vi "Module Pre-Build.vi"(6 "action":enum16{"nothing", "pre-build", "post-build"}(ring), 7 "Post-build parameters":T8 {"Build Version Info"."Build Date/Time" format="%<%H:%M:%S\n%d/%m/%Y>T"}, 8 "error in":errorcluster, 11 "Build Parameters in":T1={"Build File"=path "", "File Format Version"=0, "Build Parameters v0.0"={"Project Root"=path "", "Build Root"=path "", "Source Root"=path "", "Namespace"="", "Overwrite Existing Files?"=FALSE, "Top Level VIs"=[], "Dynamic VIs"=[], "Exclude Lib Dirs from Build (None)"=[], "Destinations"=[]}, "Extra Parameters v1.0"={"Log File"=path "", "Include Hidden VIs"=FALSE, "Include Help Files"=FALSE, "Help File Dir"=path "", "Include Shared Libs"=TRUE, "Shared Lib Dir"=path "", "Include External Subrs"=TRUE, "External Subr Dir"=path "", "Support Files"=[], "EXE Icon File"=path "", "NewBuildRootDir"=FALSE, "UnsavedChangesMsgBox"=FALSE, "Ambiguous VIs Dest Dir"=path "", "Pre-build VI"=path "", "Post-build VI"=path "", "Revision File"=path "", "Version VI Name"="", "Version Ctrl Name"="", "Default Password"="", "RemovePolyVIsAndTDs"=FALSE, "Call-Back VIs"=[], "Allow CBVI & BH overlap"=FALSE, "Namespace convention"=enum."OpenG (suffix)", "Exe.AppFlags"=0, "Exe.LVRT Res Flags"=0}, "VI Property Specs"=[]} {"File Format Version" format="%.0x"; "Extra Parameters v1.0"."Exe.LVRT Res Flags" format="%.0x"; "Extra Parameters v1.0"."Exe.AppFlags" format="%.0x"}) -> (0 "error out":errorcluster, 1 "error type":enum16{"fatal", "non-fatal", "warning"}(ring), 3 "Build Parameters out":T1={"Build File"=path "", "File Format Version"=0, "Build Parameters v0.0"={"Project Root"=path "", "Build Root"=path "", "Source Root"=path "", "Namespace"="", "Overwrite Existing Files?"=FALSE, "Top Level VIs"=[], "Dynamic VIs"=[], "Exclude Lib Dirs from Build (None)"=[], "Destinations"=[]}, "Extra Parameters v1.0"={"Log File"=path "", "Include Hidden VIs"=FALSE, "Include Help Files"=FALSE, "Help File Dir"=path "", "Include Shared Libs"=TRUE, "Shared Lib Dir"=path "", "Include External Subrs"=TRUE, "External Subr Dir"=path "", "Support Files"=[], "EXE Icon File"=path "", "NewBuildRootDir"=FALSE, "UnsavedChangesMsgBox"=FALSE, "Ambiguous VIs Dest Dir"=path "", "Pre-build VI"=path "", "Post-build VI"=path "", "Revision File"=path "", "Version VI Name"="", "Version Ctrl Name"="", "Default Password"="", "RemovePolyVIsAndTDs"=FALSE, "Call-Back VIs"=[], "Allow CBVI & BH overlap"=FALSE, "Namespace convention"=enum."OpenG (suffix)", "Exe.AppFlags"=0, "Exe.LVRT Res Flags"=0}, "VI Property Specs"=[]} {"File Format Version" format="%.0x"; "Extra Parameters v1.0"."Exe.LVRT Res Flags" format="%.0x"; "Extra Parameters v1.0"."Exe.AppFlags" format="%.0x"})   [LabVIEW 2011]
doc: "Use this VI Template to create a custom Pre-/Post-Build VI."
uses:
  <userlib>/_OpenG.lib/builder_api/ogb_api.llb/Post-build Actual Parameters__ogb_api.ctl
  <userlib>/_OpenG.lib/builder_api/ogb_api.llb/VI Build Info__ogb_api.ctl
  <userlib>/_OpenG.lib/builder_api/ogb_api.llb/Non-VI Resource Copy Info__ogb_api.ctl
  <userlib>/_OpenG.lib/builder_api/ogb_api.llb/Link Type - Enum__ogb_api.ctl
  <userlib>/_OpenG.lib/builder_api/ogb_api.llb/Version Info Cluster__ogb_api.ctl
  <userlib>/_OpenG.lib/builder_api/ogb_api.llb/Build Parameters__ogb_api.ctl
  <userlib>/_OpenG.lib/builder_api/ogb_api.llb/Build Parameters Cluster v0.0__ogb_api.ctl
  <userlib>/_OpenG.lib/builder_api/ogb_api.llb/Source Dir and Destination Cluster__ogb_api.ctl
  <userlib>/_OpenG.lib/builder_api/ogb_api.llb/Extra Build Parameters Cluster v1.0__ogb_api.ctl
  <userlib>/_OpenG.lib/builder_api/ogb_api.llb/Support Files Info Cluster__ogb_api.ctl
  <userlib>/_OpenG.lib/builder_api/ogb_api.llb/Namespasing Convention__ogb_api.ctl
  <userlib>/_OpenG.lib/builder_api/ogb_api.llb/VI Property Specifiers Info Cluster__ogb_api.ctl
  <userlib>/_OpenG.lib/file/file.llb/Append Path to Root if Relative - Scalar__ogtk.vi
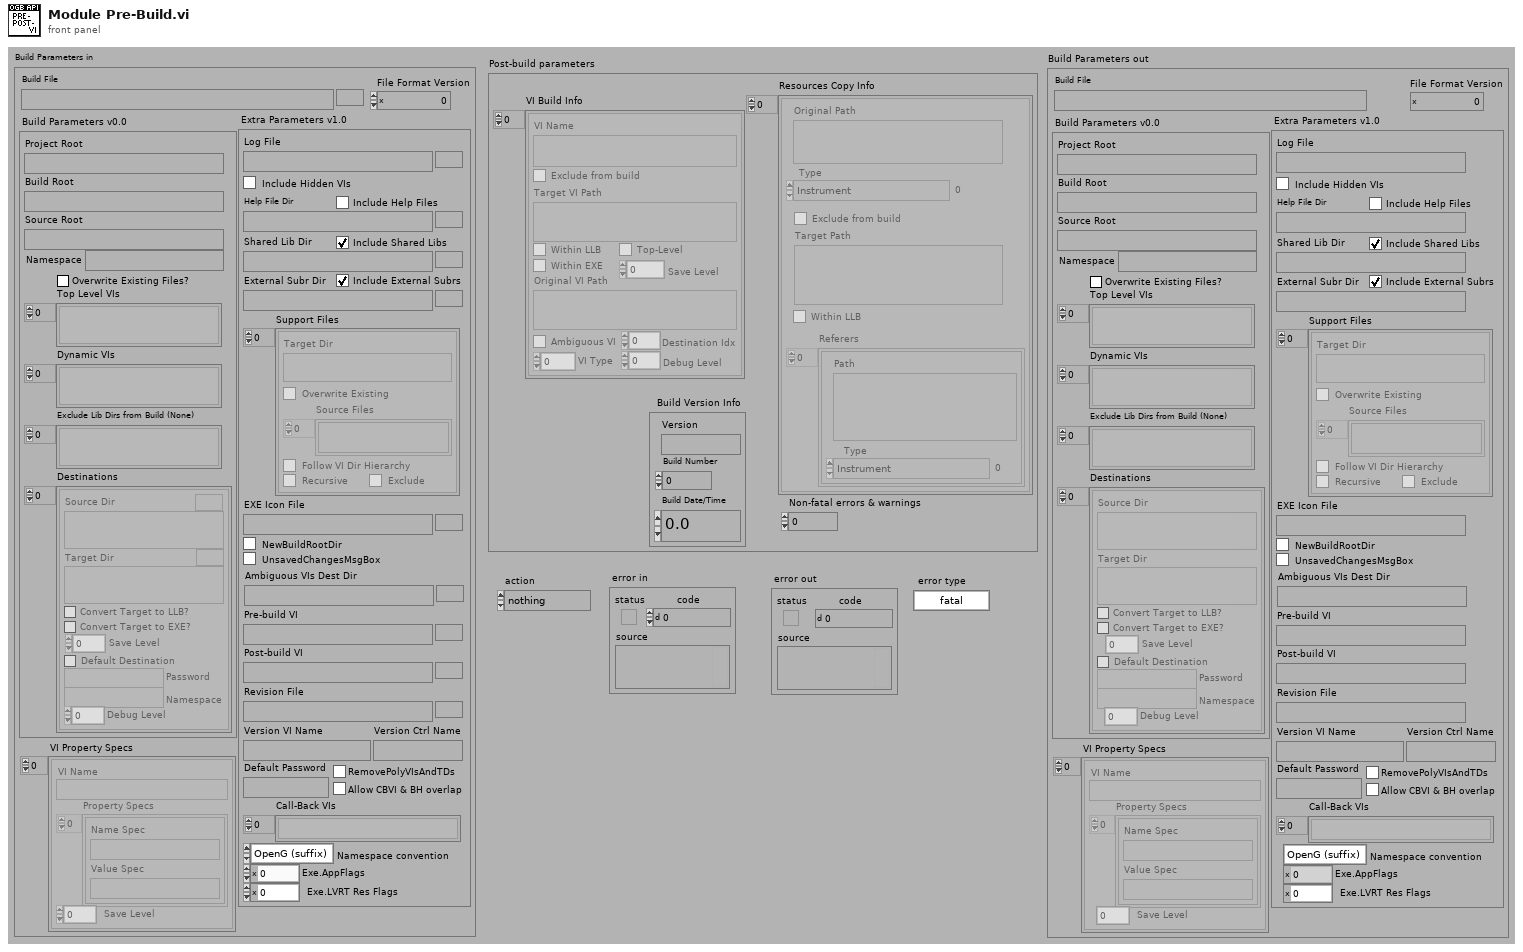
[diagram p1: front panel]
types:
  T1 = typedef "Build Parameters__ogb_api.ctl" = cluster{"Build File":path, "File Format Version":u32, "Build Parameters v0.0":T2, "Extra Parameters v1.0":T4, "VI Property Specs":T7[]}
  T2 = typedef "Build Parameters Cluster v0.0__ogb_api.ctl" = cluster{"Project Root":path, "Build Root":path, "Source Root":path, "Namespace":string, "Overwrite Existing Files?":bool, "Top Level VIs":path[], "Dynamic VIs":path[], "Exclude Lib Dirs from Build (None)":path[], "Destinations":T3[]}
  T3 = typedef "Source Dir and Destination Cluster__ogb_api.ctl" = cluster{"Source Dir":path, "Target Dir":path, "Convert Target to LLB?":bool, "Convert Target to EXE?":bool, "Save Level":i32, "Default Destination":bool, "Password":string, "Namespace":string, "Debug Level":i32}
  T4 = typedef "Extra Build Parameters Cluster v1.0__ogb_api.ctl" = cluster{"Log File":path, "Include Hidden VIs":bool, "Include Help Files":bool, "Help File Dir":path, "Include Shared Libs":bool, "Shared Lib Dir":path, "Include External Subrs":bool, "External Subr Dir":path, "Support Files":T5[], "EXE Icon File":path, "NewBuildRootDir":bool, "UnsavedChangesMsgBox":bool, "Ambiguous VIs Dest Dir":path, "Pre-build VI":path, "Post-build VI":path, "Revision File":path, "Version VI Name":string, "Version Ctrl Name":string, "Default Password":string, "RemovePolyVIsAndTDs":bool, "Call-Back VIs":path[], "Allow CBVI & BH overlap":bool, "Namespace convention":T6, "Exe.AppFlags":u32, "Exe.LVRT Res Flags":i32}
  T5 = typedef "Support Files Info Cluster__ogb_api.ctl" = cluster{"Target Dir":path, "Overwrite Existing":bool, "Source Files":path[], "Follow VI Dir Hierarchy":bool, "Recursive":bool, "Exclude":bool}
  T6 = typedef "Namespasing Convention__ogb_api.ctl" = enum32{"OpenG (suffix)", "prefix", "prefix w space"}
  T7 = typedef "VI Property Specifiers Info Cluster__ogb_api.ctl" = cluster{"VI Name":string, "Property Specs":cluster{"Name Spec":string, "Value Spec":string}[], "Save Level":i32}
  T8 = typedef "Post-build Actual Parameters__ogb_api.ctl" = cluster{"VI Build Info":T9[], "Resources Copy Info":T10[], "Non-fatal errors & warnings":i32, "Build Version Info":T12}
  T9 = typedef "VI Build Info__ogb_api.ctl" = cluster{"VI Name":string, "Exclude from build":bool, "Target VI Path":path, "Within LLB":bool, "Within EXE":bool, "Top-Level":bool, "Save Level":i32, "Original VI Path":path, "Ambiguous VI":bool, "Destination Idx":i32, "VI Type":u32, "Debug Level":i32}
  T10 = typedef "Non-VI Resource Copy Info__ogb_api.ctl" = cluster{"Original Path":path, "Type":T11, "Exclude from build":bool, "Target Path":path, "Within LLB":bool, "Referers":cluster{"Path":path, "Type":T11}[]}
  T11 = typedef "Link Type - Enum__ogb_api.ctl" = enum32{"Instrument", "Control", "CIN", "External subroutine", "Shared library", "Run-time menu", "Help file", "Palette menu", "Polymorphic VI", "Library", "Library (10)"}
  T12 = typedef "Version Info Cluster__ogb_api.ctl" = cluster{"Version":string, "Build Number":u32, "Build Date/Time":dbl}
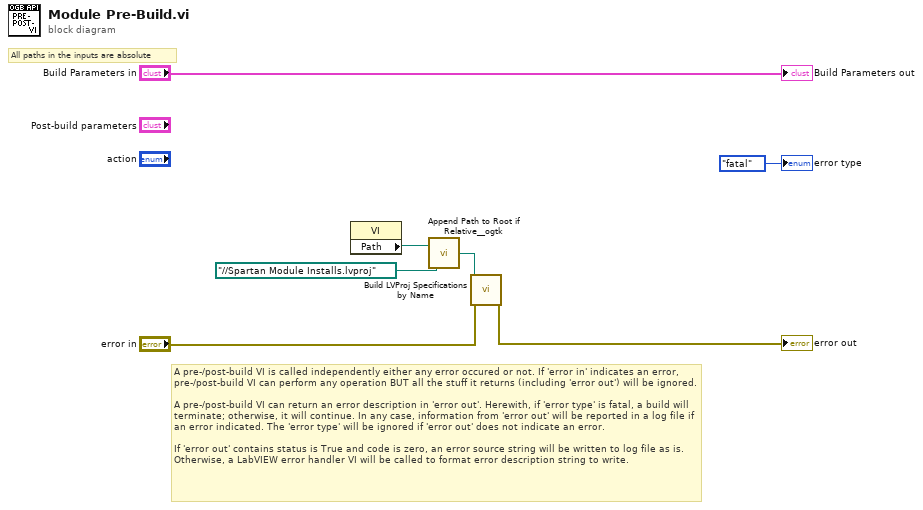
[diagram p0: block diagram]
diagram:
  # "All paths in the inputs are absolute"
  # "A pre-/post-build VI is called independently either any error occured or not. If 'error in' indicates an error, pre-/post-build VI can perform any operation BUT all the stuff it returns (including 'error out') will be ignored.\n\nA pre-/post-build VI can return an error description in 'error out'. Herewith, if 'error type' is fatal, a build will terminate; otherwise, it will continue. In any case, information from 'error out' will be reported in a log file if an error indicated. The 'error type' will be ignored if 'error out' does not indicate an error.\n\nIf 'error out' contains status is True and code is zero, an error source string will be written to log file as is. Otherwise, a LabVIEW error handler VI will be called to format error description string to write."
  n1 = property class="VI"() -> ("Path"=w3:path)  [unwired: 2 in, 2 out]
  n2 = call-poly <userlib>:"Append Path to Root if Relative__ogtk.vi"("Absolute or Relative Path"=path "../../Spartan Module Installs.lvproj" ("Path to project"), "Root Path"=w3) -> ("Absolute or Appended Path"=w1:path)
  n3 = call "Build LVProj Specifications by Name.vi"("error in (no error)"="error in", "Path to project"=w1) -> ("error out"=→"error out":errorcluster)  [unwired: 1 in, 8 out]
  "error type" <- enum16{"fatal", "non-fatal", "warning"}."fatal" ("error type")
  "Build Parameters out" <- "Build Parameters in"
